vi "Select Sweep Mode.vi"(8 "error in (no error)":errorcluster, 10 "Sweep Modes":T1, 11 "Yokogawa AQ6370D in":refnum<class "Yokogawa AQ6370D.lvclass">) -> (0 "error out":errorcluster, 3 "Yokogawa AQ6370D out":refnum<class "Yokogawa AQ6370D.lvclass">)   [LabVIEW 2018, in "Yokogawa AQ6370D.lvlib" / "Yokogawa AQ6370D.lvclass"]
uses:
  Yokogawa AQ6370D.lvclass
  PPLs/Optical Spectrum Analyzer/Parent/OSA.lvlibp/Custom Controls/enm_Sweep Modes.ctl
  Yokogawa AQ6370D.lvclass/Yokogawa AQ6370D.ctl
  PPLs/Optical Spectrum Analyzer/Parent/OSA.lvlibp/Optical Spectrum Analyzer.lvclass
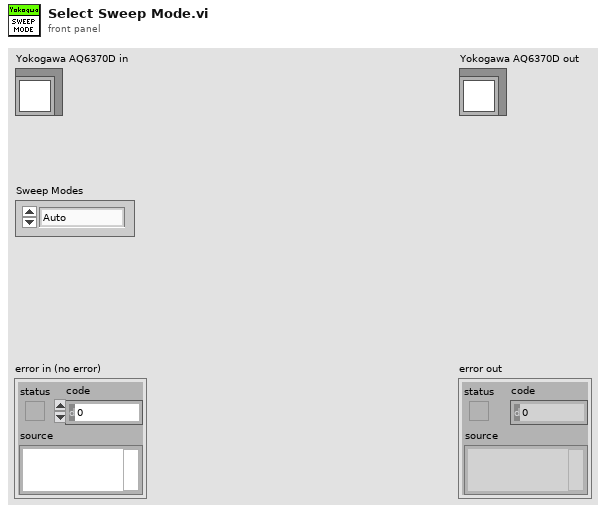
[diagram p1: front panel]
types:
  T1 = typedef "OSA.lvlibp/Optical Spectrum Analyzer.lvclass/enm_Sweep Modes.ctl" = enum16{"Auto", "Repeat", "Single", "Stop", "Segment"}
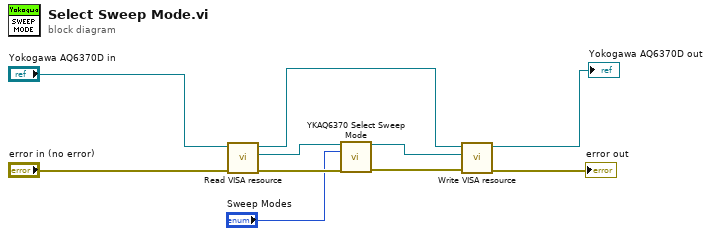
[diagram p0: block diagram]
diagram:
  n1 = call "Read VISA resource.vi"("error in (no error)"="error in (no error)", "Yokogawa AQ6370D in"="Yokogawa AQ6370D in") -> ("error out"=w5:errorcluster, "VISA resource"=w3:refnum<visa-resource-name>, "Yokogawa AQ6370D out"=w6:refnum<class "Yokogawa AQ6370D.lvclass">)  [unwired: 7 in]
  n2 = call <instrlib>:"YKAQ6370 Select Sweep Mode.vi"("VISA resource name"=w3, "Action Select (3: Stop)"="Sweep Modes", "error in (no error)"=w5) -> ("VISA resource name out"=w1:refnum<visa-resource-name>, "error out"=w4:errorcluster)  [unwired: 11 in]
  n3 = call "Write VISA resource.vi"("error in (no error)"=w4, "VISA resource"=w1, "Yokogawa AQ6370D in"=w6) -> ("error out"=→"error out":errorcluster, "Yokogawa AQ6370D out"=→"Yokogawa AQ6370D out":refnum<class "Yokogawa AQ6370D.lvclass">)  [unwired: 7 in]
